vi "Configure Interrupts.vi"(7 "I2C Channel":u8, 8 "error in (no error)":errorcluster, 10 "Interrupt Configuration":T1={"<INT CFG> INT OUT pin Logic Level"=0, "<INT CFG> Out pin Drive Type"=64, "<INT CFG> Latch Mode"=32, "<INT CFG> Latch Clear Mode"=0, "<INT CFG> INT on Data RDY"=1, "<INT CFG> Enable INT on Device RDY"=4} {"<INT CFG> Enable INT on Device RDY" items=["Enable INT on Device RDY (on PLL RDY)"=4, "Disable  INT on Device RDY"=0]; "<INT CFG> INT on Data RDY" items=["Enable  INT on  Data RDY"=1, "Disable  INT on  Data RDY"=0]; "<INT CFG> Latch Clear Mode" items=["Clear INT on Any Register Read"=16, "Status Register Read Only"=0]; "<INT CFG> Latch Mode" items=["Latch until INT Cleared"=32, "50us Pulse"=0]; "<INT CFG> Out pin Drive Type" items=["Open Drain"=64, "Push-Pull"=0]; "<INT CFG> INT OUT pin Logic Level" items=["Active Low"=128, "Active High"=0]}, 11 "LINX Resource In":T2) -> (0 "error out":errorcluster, 3 "LINX Resource Out":T2)   [LabVIEW 2014, in "LMH-LINX.lvlib" / "ITG3200.lvlib"]
uses:
  <vilib>/MakerHub/LINX/Public/Sensors/Gyroscopes/ITG3200/ITG3200.lvlib
  <vilib>/MakerHub/LINX/Private/Type Defs/LINX Ref.ctl
  <vilib>/MakerHub/LINX/Private/Type Defs/Platform.ctl
  <vilib>/MakerHub/LINX/Private/Type Defs/Interface.ctl
  <vilib>/MakerHub/LINX/Private/Device/Type Defs/LINX Device Config.ctl
  <vilib>/MakerHub/LINX/Private/Device/Type Defs/TCP Config.ctl
  <vilib>/MakerHub/LINX/Private/Device/Type Defs/Channels.ctl
  <vilib>/MakerHub/LINX/Public/Sensors/Gyroscopes/ITG3200/Controls/Int_Config.ctl
  <vilib>/MakerHub/LINX/Private/Local IO/LinxI2cWrite.vi
  <vilib>/MakerHub/LINX/Public/Utilities/Check Channel.vi
  <vilib>/MakerHub/LINX/Private/Utilties/Generate Error.vi
  <vilib>/MakerHub/LINX/LMH-LINX.lvlib
  <vilib>/MakerHub/LINX/Private/Device/Device.lvlib
panel:
  # "INPUTS"
  # "OUTPUTS"
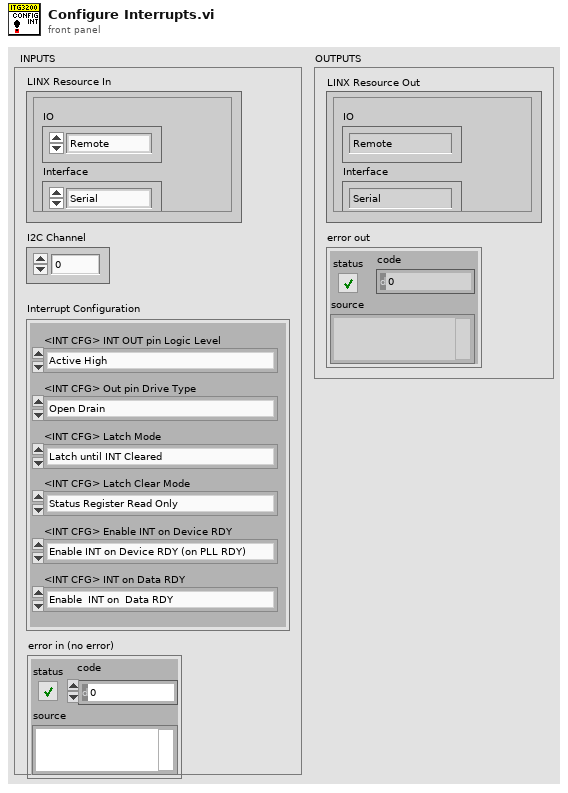
[diagram p1: front panel]
types:
  T1 = typedef "Int_Config.ctl" = cluster{"<INT CFG> INT OUT pin Logic Level":u8, "<INT CFG> Out pin Drive Type":u8, "<INT CFG> Latch Mode":u8, "<INT CFG> Latch Clear Mode":u8, "<INT CFG> INT on Data RDY":u8, "<INT CFG> Enable INT on Device RDY":u8}
  T2 = typedef "LMH-LINX.lvlib/LINX Ref.ctl" = cluster{"IO":T3, "Interface":T4, "LINX Device Config":T5}
  T3 = typedef "LMH-LINX.lvlib/Platform.ctl" = enum16{"Remote", "Local"}
  T4 = typedef "LMH-LINX.lvlib/Interface.ctl" = enum16{"Serial", "TCP"}
  T5 = typedef "LMH-LINX.lvlib/Device.lvlib/LINX Device Config.ctl" = cluster{"Interface":T4, "COM Port":refnum<visa-resource-name>, "TCP Configuration":T6, "Device Family":u8, "Device ID":u8, "Device Name":string, "TCP Ref":refnum<k5>, "Channels":T7}
  T6 = typedef "LMH-LINX.lvlib/Device.lvlib/TCP Config.ctl" = cluster{"IP Address":string, "Port":u16}
  T7 = typedef "LMH-LINX.lvlib/Channels.ctl" = cluster{"DI":u8[], "DO":u8[], "AI":u8[], "AO":u8[], "PWM":u8[], "QE":u8[], "UART":u8[], "I2C 2":u8[], "SPI":u8[], "CAN":u8[], "Servo":u8[], "AI Ref (V)":dbl, "AI Resolution (Bits)":u8, "AO Ref (V)":dbl, "AO Resolution (Bits)":u8}
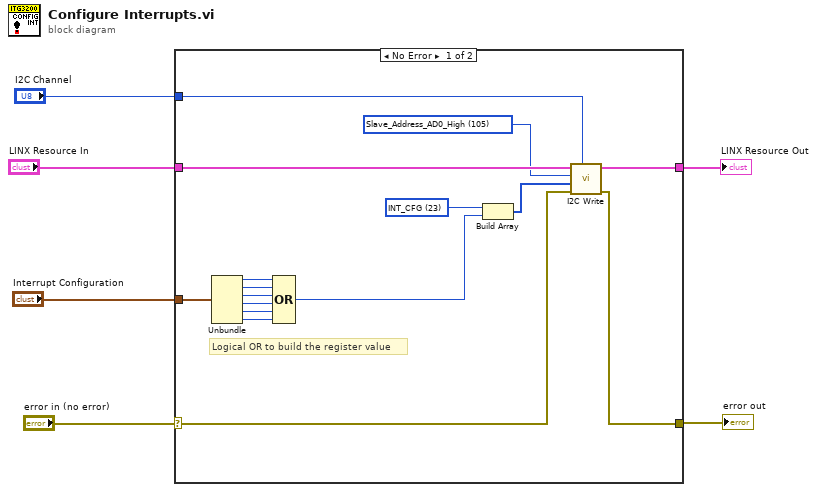
[diagram p0: block diagram]
diagram:
  n1 = case shown="No Error" "error in (no error)" {
    selector: "error in (no error)" -> [w21 w24]
    tunnel: [w7 w24] -> w5
    tunnel: "LINX Resource In" -> [w22 w23]
    tunnel: "I2C Channel" -> [w18 _]
    tunnel: [w8 w23] -> w2
    tunnel: "Interrupt Configuration" -> [w16 _]
    frame No Error {
      w20 = u8 23 items=["WHO_AM_I"=0, "SMPLRT_DIV"=21, "DLPF_FS"=22, "INT_CFG"=23, "INT_STATUS"=26, "TEMP_OUT_H"=27, "TEMP_OUT_L"=28, "GYRO_XOUT_H"=29, "GYRO_XOUT_L"=30, "GYRO_YOUT_H"=31, "GYRO_YOUT_L"=32, "GYRO_ZOUT_H"=33, "GYRO_ZOUT_L"=34, "PWR_MGM"=62] ("Register Map")
      w17 = u8 105 items=["Slave_Address_AD0_Low"=104, "Slave_Address_AD0_High"=105] ("Slave Addresses")
      # "Logical OR to build the register value"
      n2 = Unbundle(w16) -> ("<INT CFG> INT OUT pin Logic Level"=w15:u8, "<INT CFG> Out pin Drive Type"=w14:u8, "<INT CFG> Latch Mode"=w13:u8, "<INT CFG> Latch Clear Mode"=w12:u8, "<INT CFG> INT on Data RDY"=w11:u8, "<INT CFG> Enable INT on Device RDY"=w10:u8)
      n3 = Compound Arithmetic op=OR(w15, w14, w13, w12, w11, w10) -> (w9:u8)
      n4 = Build Array(w20, w9) -> (w19:u8[])
      n5 = call <vilib>:"I2C Write.vi"("I2C Channel"=w18, "Error In"=w21, "Data"=w19, "I2C Slave Address (0)"=w17, "LINX Resource"=w22) -> ("Error Out"=w7:errorcluster, "LINX Resource"=w8:T2)  [unwired: 5 in]
    }
    frame Error {
    }
  }
  "error out" <- w5
  "LINX Resource Out" <- w2
